vi "Get Name.vi"(8 "error in (no error)":errorcluster, 11 "reference Class in":refnum<class "Reference Class.lvclass">) -> (0 "error out":errorcluster, 2 "name":string, 3 "reference Class out":refnum<class "Reference Class.lvclass">)   [LabVIEW 2023, in "Reference Class.lvclass"]
doc: "Get \"name.\""
uses:
  Reference Class.lvclass
  Reference Class.lvclass/Reference Class.ctl
  SimpleClass/Simple Class.lvclass
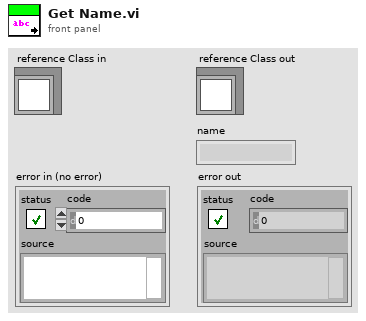
[diagram p1: front panel]
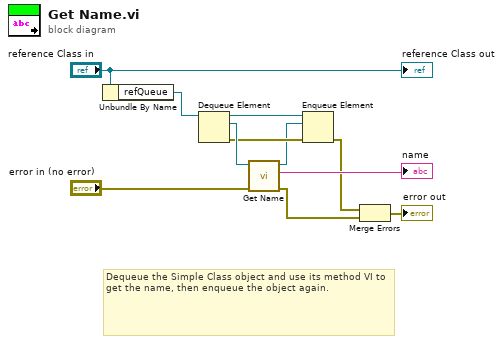
[diagram p0: block diagram]
diagram:
  # "Dequeue the Simple Class object and use its method VI to get the name, then enqueue the object again."
  n1 = Unbundle By Name("reference Class in") -> ("refQueue"=w8:refnum<queue>)
  n2 = Dequeue Element(queue=w8) -> (queue out=w6:refnum<queue>, element=w7:refnum<class "Simple Class.lvclass">, error out=w5:errorcluster)  [unwired: 2 in, 1 out]
  n3 = call "Get Name.vi"("error in (no error)"="error in (no error)", "simple Class in"=w7) -> ("error out"=w1:errorcluster, "name"=→"name":string, "simple Class out"=w4:refnum<class "Simple Class.lvclass">)  [unwired: 7 in]
  n4 = Enqueue Element(queue=w6, element=w4, error in (no error)=w5) -> (error out=w2:errorcluster)  [unwired: 1 in, 2 out]
  n5 = Merge Errors(w2, w1) -> (→"error out":errorcluster)
  "reference Class out" <- "reference Class in"
